vi "Initialize.vi"(6 "error in":errorcluster, 9 "NI MAX name":string) -> (0 "error out":errorcluster, 3 "VISA resource name out":refnum<visa-resource-name>)   [LabVIEW 2023, in "Aim TTi 1908P DMM.lvlib"]
uses:
  Aim TTi 1908P DMM.lvlib
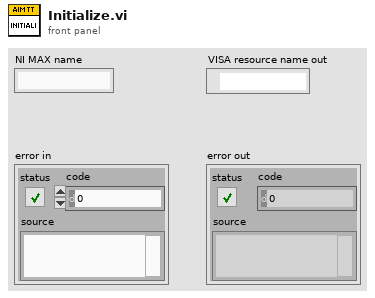
[diagram p1: front panel]
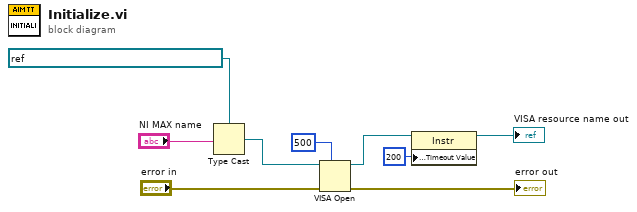
[diagram p0: block diagram]
diagram:
  n1 = Type Cast(type=refnum<visa-resource-name> "TCPIP0::192.168.0.11::9221::SOCKET" ("VISA resource name"), x="NI MAX name") -> (*(type *) &x=w5:refnum<visa-resource-name>)
  n2 = VISA Open(timeout (0)=u32 500 ("VISA Open timeout (0)"), error in (no error)="error in", VISA resource name=w5) -> (VISA resource name=w2:refnum<visa-resource-name>, error out=→"error out":errorcluster)  [unwired: 2 in]
  n3 = property class="Instr"(reference=w2, "General Settings:Timeout Value"=u32 200) -> (reference out=→"VISA resource name out":refnum<visa-resource-name>)  [unwired: 1 in, 1 out]
